vi "ATS_SetCaptureClock.vi"(10 "Clock":T1 {"ClckEdge" items=["Rising", "Falling"]; "ClckRate" items=["1 kS/s", "2 kS/s", "5 kS/s", "10 kS/s", "20 kS/s", "50 kS/s", "100 kS/s", "200 kS/s", "500 kS/s", "1 MS/s", "2 MS/s", "5 MS/s", "10 MS/s", "20 MS/s", "25 MS/s", "50 MS/s", "100 MS/s", "125 MS/s", "200 MS/s", "250 MS/s", "500 MS/s", "1 GS/s"]}, 11 "DeviceIn":i32) -> (0 "Return Code":u32, 2 "Clock_Value (s)":dbl format="%.2p", 3 "DeviceOut":i32)   [LabVIEW 2014]
doc: "_____AlazarTech, Scope_____\n\nConfigure the capture clock circuitry."
uses:
  ATS_ctl/Clock.ctl
  ATS_ctl/ClockSource.ctl
  ATS_ctl/ClockRate.ctl
  ATS_ctl/ClockEdge.ctl
  ATS_ctl/ATS_Global_Ctrl.ctl
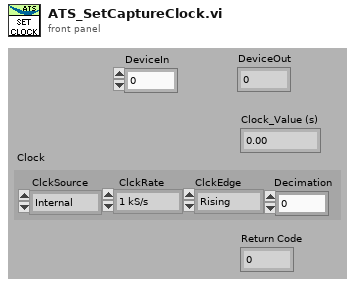
[diagram p1: front panel]
types:
  T1 = typedef "Clock.ctl" = cluster{"ClckSource":T2, "ClckRate":T3, "ClckEdge":T4, "Decimation":u32}
  T2 = typedef "ClockSource.ctl" = enum16{"Internal", "External", "Medium Ext.", "Slow Ext.", "Ext. AC", "Ext. DC", "Ext. (PLL)"}
  T3 = typedef "ClockRate.ctl" = u32
  T4 = typedef "ClockEdge.ctl" = u16
  T5 = typedef "ATS_Global_Ctrl.ctl" = enum16{"Init_Device", "Clear_ALL", "Set", "Get"}
  T6 = typedef "ATS_Set_Value.ctl" = cluster{"Clock (s)":dbl, "RangeA (v)":dbl, "RangeB (v)":dbl, "Ranges (v)":dbl[]}
  T7 = typedef "ATS_Global_4Ch.ctl" = cluster{"Record":T8, "Clock":T1, "Inputs":T9, "Trigger":T15}
  T8 = typedef "Record.ctl" = cluster{"Count":u32, "Presize":u32, "Length":u32}
  T9 = typedef "ATS_InputArray.ctl" = T10[]
  T10 = typedef "InputCtrl.ctl" = cluster{"Coupling":T11, "Range":T12, "Impedance":T13, "Bandwidth":T14}
  T11 = typedef "Coupling.ctl" = enum16{"AC", "DC"}
  T12 = typedef "Range.ctl" = u32
  T13 = typedef "Impedance.ctl" = enum16{"1M ohms", "50 ohms"}
  T14 = typedef "Bandwidth.ctl" = enum16{"Full Bandwidth", "Reduce Bandwidth"}
  T15 = typedef "ATS_Trigger_4Ch.ctl" = cluster{"TrigOperation":T16, "Timeout (s)":dbl, "Trig. Delay":u32, "Engine X":T17, "Engine Y":T17, "ExtTrigControl":T19}
  T16 = typedef "TriggerOperation.ctl" = enum16{"Only X", "Only Y", "X or Y", "X and Y", "X xor Y", "X and not Y", "not X and Y"}
  T17 = typedef "ATS_TriggerEngine_4Ch.ctl" = cluster{"Source":T18, "Slope":enum32{"Positive", "Negative"}, "Level":u32}
  T18 = typedef "ATS_TriggerSource_4Ch.ctl" = enum32{"Chan_A", "Chan_B", "External", "Disable", "Chan_C", "Chan_D"}
  T19 = typedef "ExtTrigger.ctl" = cluster{"Coupling":T11, "Range":T20}
  T20 = typedef "ExtTrigRange.ctl" = enum16{"1 V", "5 V", "TTL"}
  T21 = typedef "Device_Info.ctl" = cluster{"Handle":u32, "Board":string, "CPLD":string, "MemorySize":u32, "SampleSize":u8, "ID":i32, "High_Memory":bool, "Chan/Board":u8}
  T22 = typedef "ATS_Card_Spec.ctl" = cluster{"Name":string, "Rate":string[], "Range":string[], "RangeLim(50)":u32, "Bandwidth":bool}
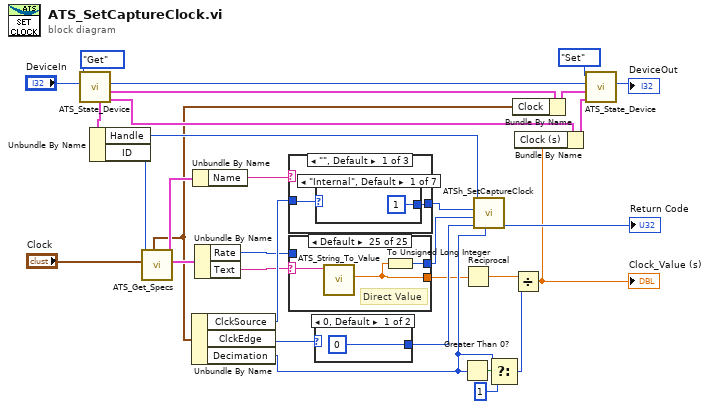
[diagram p0: block diagram]
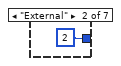
[diagram p2: hidden frame]
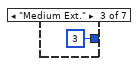
[diagram p3: hidden frame]
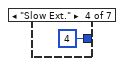
[diagram p4: hidden frame]
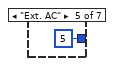
[diagram p5: hidden frame]
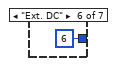
[diagram p6: hidden frame]
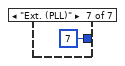
[diagram p7: hidden frame]
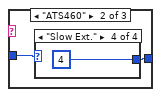
[diagram p8: hidden frame]
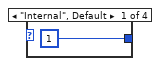
[diagram p9: hidden frame]
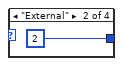
[diagram p10: hidden frame]
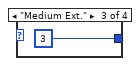
[diagram p11: hidden frame]
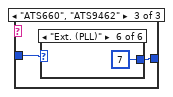
[diagram p12: hidden frame]
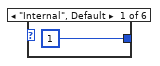
[diagram p13: hidden frame]
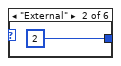
[diagram p14: hidden frame]
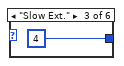
[diagram p15: hidden frame]
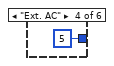
[diagram p16: hidden frame]
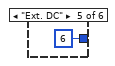
[diagram p17: hidden frame]
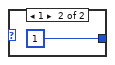
[diagram p18: hidden frame]
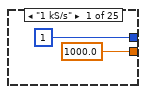
[diagram p19: hidden frame]
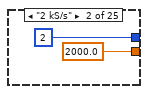
[diagram p20: hidden frame]
diagram:
  n1 = call "ATS_State_Device.vi"("DeviceIn"="DeviceIn", "ATS_GBL_Ctrl"=ATS_Global_Ctrl."Get") -> ("Ref_Out"=w20:T6, "SetupOut"=w22:T7, "DeviceOut"=w28:i32, "DevInfo_Out"=w19:T21)  [unwired: 4 in, 2 out]
  n2 = Unbundle By Name(w19) -> ("Handle"=w24:u32, "ID"=w16:i32)
  n3 = call "ATS_Get_Specs.vi"("Clock_Input"="Clock", "ID"=w16) -> ("Rate_Out"=w14:cluster{"Text":string, "Rate":u32}, "Card_Spec"=w13:T22, "Clock_Output"=w10:T1)  [unwired: 5 in, 2 out]
  n4 = Unbundle By Name(w10) -> ("ClckSource"=w26:T2, "ClckEdge"=w25:T4, "Decimation"=w5:u32)
  n5 = Unbundle By Name(w13) -> ("Name"=w12:string)
  n6 = Unbundle By Name(w14) -> ("Rate"=w9:u32, "Text"=w15:string)
  n7 = case shown="\"\", Default" w12 {
    tunnel: [w33 w43 w49] -> w31
    tunnel: w26 -> [w34 w42 w48]
    frame "", Default {
      n8 = case shown="\"Internal\", Default" w34 {
        tunnel: [u32 1 ("Operation") u32 2 ("Operation") u32 3 ("Operation") u32 4 ("Operation") u32 5 ("Operation") u32 6 ("Operation") u32 7 ("Operation")] -> w33
        frame "Internal", Default {
        }
        frame "External" {
        }
        frame "Medium Ext." {
        }
        frame "Slow Ext." {
        }
        frame "Ext. AC" {
        }
        frame "Ext. DC" {
        }
        frame "Ext. (PLL)" {
        }
      }
    }
    frame "ATS460" {
      n9 = case shown="\"Slow Ext.\"" w42 {
        tunnel: [u32 1 ("Operation") u32 2 ("Operation") u32 3 ("Operation") u32 4 ("Operation")] -> w43
        frame "Internal", Default {
        }
        frame "External" {
        }
        frame "Medium Ext." {
        }
        frame "Slow Ext." {
        }
      }
    }
    frame "ATS660", "ATS9462" {
      n10 = case shown="\"Ext. (PLL)\"" w48 {
        tunnel: [u32 1 ("Operation") u32 2 ("Operation") u32 4 ("Operation") u32 5 ("Operation") u32 6 ("Operation") u32 7 ("Operation")] -> w49
        frame "Internal", Default {
        }
        frame "External" {
        }
        frame "Slow Ext." {
        }
        frame "Ext. AC" {
        }
        frame "Ext. DC" {
        }
        frame "Ext. (PLL)" {
        }
      }
    }
  }
  n11 = case shown="Default" w15 {
    selector: w15 -> [_ _ _ _ _ _ _ _ _ _ _ _ _ _ _ _ _ _ _ _ _ _ _ _ w106]
    tunnel: [u32 1 ("Operation") u32 2 ("Operation") u32 4 ("Operation") u32 8 ("Operation") u32 10 ("Operation") u32 12 ("Operation") u32 14 ("Operation") u32 16 ("Operation") u32 18 ("Operation") u32 20 ("Operation") u32 24 ("Operation") u32 26 ("Operation") u32 28 ("Operation") u32 30 ("Operation") u32 33 ("Operation") u32 34 ("Operation") u32 36 ("Operation") u32 37 ("Operation") u32 38 ("Operation") u32 39 ("Operation") u32 40 ("Operation") u32 43 ("Operation") u32 48 ("Operation") u32 53 ("Operation") w105] -> w8
    tunnel: [1000.0 2000.0 5000.0 10000.0 20000.0 50000.0 100000.0 200000.0 500000.0 1000000.0 2000000.0 5000000.0 10000000.0 20000000.0 25000000.0 50000000.0 100000000.0 125000000.0 160000000.0 180000000.0 200000000.0 250000000.0 500000000.0 1000000000.0 w104] -> w3
    tunnel: w9 -> [_ _ _ _ _ _ _ _ _ _ _ _ _ _ _ _ _ _ _ _ _ _ _ _ _]
    frame "1 kS/s" {
    }
    frame "2 kS/s" {
    }
    frame "5 kS/s" {
    }
    frame "10 kS/s" {
    }
    frame "20 kS/s" {
    }
    frame "50 kS/s" {
    }
    frame "100 kS/s" {
    }
    frame "200 kS/s" {
    }
    frame "500 kS/s" {
    }
    frame "1 MS/s" {
    }
    frame "2 MS/s" {
    }
    frame "5 MS/s" {
    }
    frame "10 MS/s" {
    }
    frame "20 MS/s" {
    }
    frame "25 MS/s" {
    }
    frame "50 MS/s" {
    }
    frame "100 MS/s" {
    }
    frame "125 MS/s" {
    }
    frame "160 MS/s" {
    }
    frame "180 MS/s" {
    }
    frame "200 MS/s" {
    }
    frame "250 MS/s" {
    }
    frame "500 MS/s" {
    }
    frame "1 GS/s" {
    }
    frame Default {
      # "Direct Value"
      n12 = call "ATS_String_To_Value.vi"("String_In"=w106) -> ("Value_Out"=w104:dbl)  [unwired: 5 in, 1 out]
      n13 = To Unsigned Long Integer(number=w104) -> (unsigned 32bit integer=w105:u32)
    }
  }
  n14 = case shown="0, Default" w25 {
    tunnel: [u32 0 ("Operation") u32 1 ("Operation")] -> w7
    frame 0, Default {
    }
    frame 1 {
    }
  }
  n15 = Greater Than 0?(x=w5) -> (x > 0?=w6:bool)
  n16 = Reciprocal(x=w3) -> (1/x=w21:dbl)
  n17 = call "ATSh_SetCaptureClock.vi"("Decimation"=w5, "Edge"=w7, "Rate"=w8, "Source"=w31, "Handle"=w24) -> ("Return"=→"Return Code":u32)  [unwired: 5 in, 1 out]
  n18 = Select(t=w5, s=w6, f=u32 1) -> (s? t:f=w1:u32)
  n19 = Bundle By Name(cluster=w22, "Clock"=w10) -> (w23:T7)
  n20 = Divide(x=w21, y=w1) -> (x/y=w2:dbl)
  "Clock_Value (s)" <- w2
  n21 = Bundle By Name(cluster=w20, "Clock (s)"=w2) -> (w18:T6)
  n22 = call "ATS_State_Device.vi"("Ref_In"=w18, "SetupIn"=w23, "DeviceIn"=w28, "ATS_GBL_Ctrl"=ATS_Global_Ctrl."Set") -> ("DeviceOut"=→"DeviceOut":i32)  [unwired: 2 in, 5 out]
